vi "Test_Skew.vi"() -> ()   [LabVIEW 2020]
uses:
  <vilib>/vision/NI_Vision_Development_Module.lvlib
panel:
  in  "Sample":u16(ring) items=["Visualize", "Benchmark"]
  in  "Test Skewer":T1(ring)
  in  "Continious Skewing":bool
  in  "Calculation mode":enum16{"Single core", "2x cores", "4x cores"}(ring)
  out "Elapsed time [ms]":u32
  in  "Refresh Image":bool
  in  "Skew on X":bool
  in  "Share Angle":u16 max=89 step=1
  in  "stop":bool
  out "Image":T2(plugin-control)
  # "0, 1 ... 89"
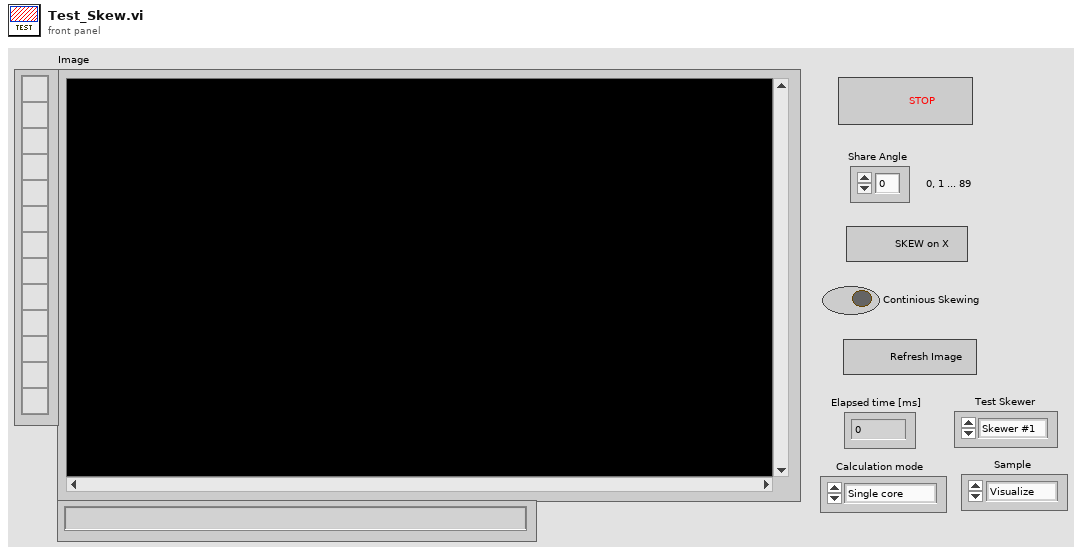
[diagram p1: front panel]
types:
  T1 = enum16{"Skewer #1", "Skewer #2", "Skewer #3", "Skewer #4", "Skewer #5"}
  T2 = typedef "IMAQ Image.ctl" = refnum<image>
  T3 = typedef "Image Type" = u32
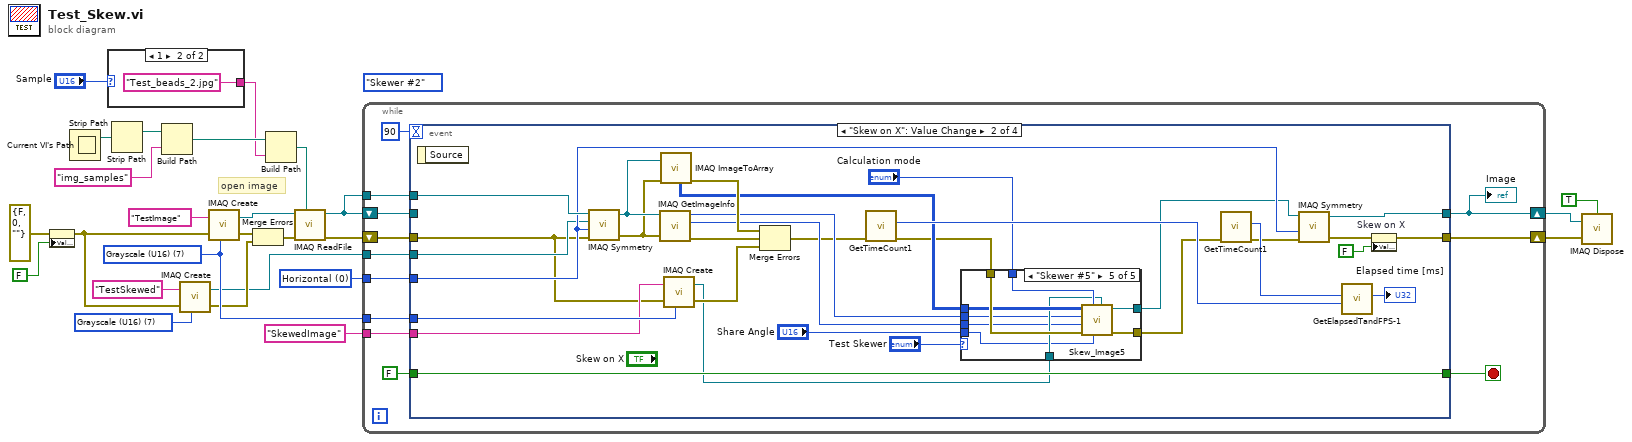
[diagram p0: block diagram]
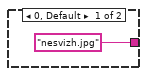
[diagram p2: hidden frame]
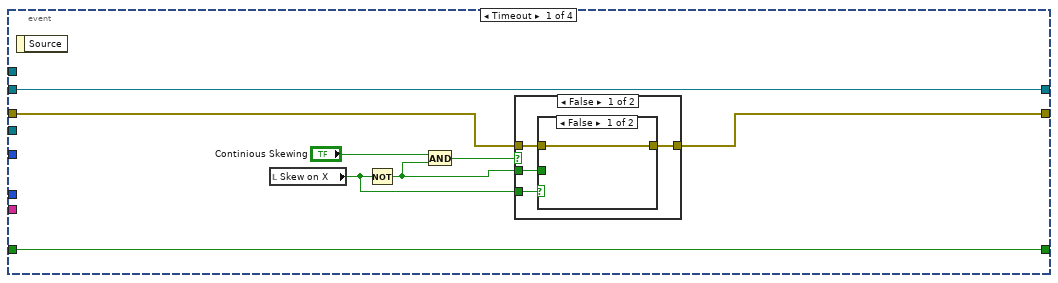
[diagram p3: hidden frame]
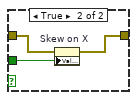
[diagram p4: hidden frame]
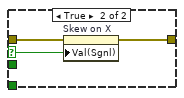
[diagram p5: hidden frame]
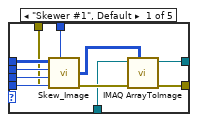
[diagram p6: hidden frame]
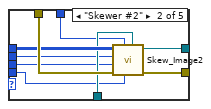
[diagram p7: hidden frame]
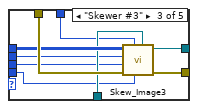
[diagram p8: hidden frame]
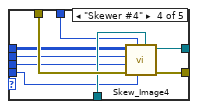
[diagram p9: hidden frame]
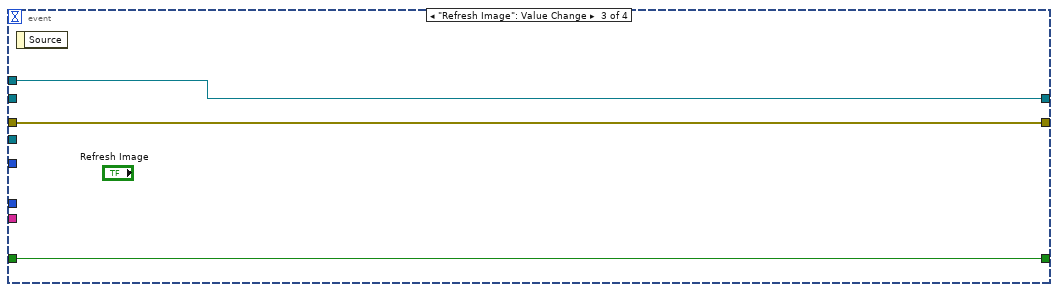
[diagram p10: hidden frame]
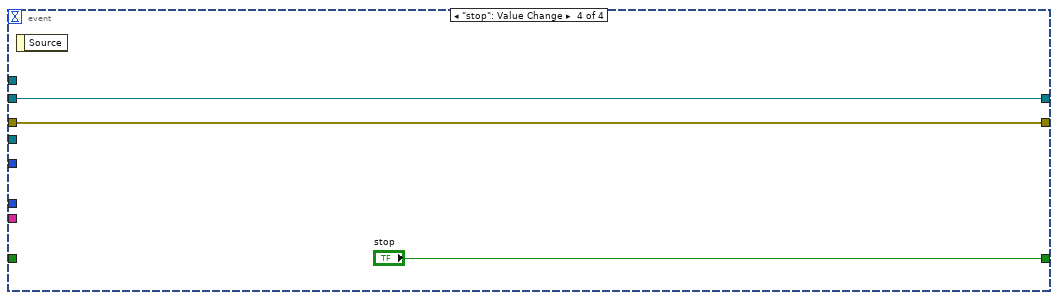
[diagram p11: hidden frame]
diagram:
  (unwired) enum16{"Skewer #1", "Skewer #2"}."Skewer #2"
  w11 = T3 7 items=["Grayscale (U8)", "Grayscale (I16)", "Grayscale (SGL)", "Complex (CSG)", "RGB (U32)", "HSL (U32)", "RGB (U64)", "Grayscale (U16)"] ("Image Type")
  w13 = u32 0 items=["Horizontal", "Vertical", "Central", "1st Diagonal", "2nd Diagonal"] ("Type of Symmetry")
  w17 = T3 7 items=["Grayscale (U8)", "Grayscale (I16)", "Grayscale (SGL)", "Complex (CSG)", "RGB (U32)", "HSL (U32)", "RGB (U64)", "Grayscale (U16)"] ("Image Type")
  # "open image"
  n1 = property on="Continious Skewing" class="Bool (strict)"(error in=errorcluster {"status"=FALSE, "code"=0, "source"=""} ("error in (no error)"), "Value"=FALSE ("Continious Skewing")) -> (error out=w4:errorcluster)  [unwired: 1 in, 1 out]
  n2 = Current VI's Path() -> (path=w27:path)
  n3 = Strip Path(path=w27) -> (stripped path=w23:path)  [unwired: 1 out]
  n4 = case shown="1" "Sample" {
    tunnel: ["nesvizh.jpg" ("name or relative path") "Test_beads_2.jpg" ("name or relative path")] -> w1
    frame 0, Default {
    }
    frame 1 {
    }
  }
  n5 = Strip Path(path=w23) -> (stripped path=w22:path)  [unwired: 1 out]
  n6 = Build Path(base path=w22, name or relative path="img_samples") -> (appended path=w20:path)
  n7 = call "IMAQ Create"("Image Name"="TestSkewed", "Image Type"=w11, "error in (no error)"=w4) -> ("New Image"=w7:T2, "error out"=w8:errorcluster)  [unwired: 2 in]
  n8 = call "IMAQ Create"("Image Name"="TestImage", "Image Type"=w17, "error in (no error)"=w4) -> ("New Image"=w24:T2, "error out"=w10:errorcluster)  [unwired: 2 in]
  n9 = Merge Errors(w10, w8) -> (w9:errorcluster)
  n10 = Build Path(base path=w20, name or relative path=w1) -> (appended path=w26:path)
  n11 = call "IMAQ ReadFile"("File Path"=w26, "error in (no error)"=w9, "Image"=w24) -> ("error out"=w19:errorcluster, "Image Out"=w15:T2)  [unwired: 4 in, 3 out]
  n12 = while {
    shift-right: [w39] -> w18
    shift-left: w19 -> [w40]
    tunnel: w17 -> [w35]
    shift-right: [w34] -> w14
    shift-left: w15 -> [w38]
    tunnel: w15 -> [w33]
    tunnel: w13 -> [w32]
    tunnel: w7 -> [w31]
    tunnel: "SkewedImage" ("Image Name") -> [w30]
    stop <- w36 stop-if-true
    n13 = event shown="[1] \"Skew on X\": Value Change" {
      selector: _ -> [_ _ _ _]
      dyn-events: _ -> [_ _ _ _]
      timeout: 90 -> [_ _ _ _]
      tunnel: w40 -> [w47 w67 w139 w143]
      tunnel: [w46 w72 w139 w143] -> w39
      tunnel: [w48 w91 w138 "stop"] -> w36
      tunnel: w38 -> [w49 _ _ w141]
      tunnel: [w49 w80 w140 w141] -> w34
      tunnel: FALSE ("stop") -> [w48 w91 w138 _]
      tunnel: w35 -> [_ w90 _ _]
      tunnel: w33 -> [_ w86 w140 _]
      tunnel: w32 -> [_ w83 _ _]
      tunnel: w31 -> [_ w82 _ _]
      tunnel: w30 -> [_ w81 _ _]
      event Timeout {
        n14 = event-data() -> ()  [unwired: 1 in, 1 out]
        n15 = local read "Skew on X"() -> (w43:bool)
        n16 = Not(x=w43) -> (.not. x?=w42:bool)
        n17 = And(x="Continious Skewing", y=w42) -> (x .and. y?=w44:bool)
        n18 = case shown="False" w44 {
          selector: w44 -> [_ w58]
          tunnel: w47 -> [w52 w60]
          tunnel: [w51 w59] -> w46
          tunnel: w43 -> [w53 _]
          tunnel: w42 -> [w50 _]
          frame False {
            n19 = case shown="False" w53 {
              tunnel: w52 -> [w54 w57]
              tunnel: [w54 w56] -> w51
              tunnel: w50 -> [_ w55]
              frame False {
              }
              frame True {
                n20 = property on="Skew on X" class="Bool (strict)"(error in=w57, "Value"=w55) -> (error out=w56:errorcluster)  [unwired: 1 in, 1 out]
              }
            }
          }
          frame True {
            n21 = property on="Skew on X" class="Bool (strict)"(error in=w60, "Val(Sgnl)"=w58) -> (error out=w59:errorcluster)  [unwired: 1 in, 1 out]
          }
        }
      }
      event "Skew on X": Value Change {
        n22 = event-data() -> ()  [unwired: 1 in, 1 out]
        n23 = call "IMAQ Symmetry"("error in (no error)"=w67, "Type of Symmetry"=w83, "Image Dst"=w82, "Image Src"=w86) -> ("error out"=w84:errorcluster, "Image Dst Out"=w85:T2)  [unwired: 1 in]
        n24 = call "IMAQ GetImageInfo"("error in (no error)"=w84, "Image"=w85) -> ("error out"=w89:errorcluster, "Y Resolution"=w73:i32, "X Resolution"=w74:i32)  [unwired: 2 in, 5 out]
        n25 = call "IMAQ ImageToArray"("error in (no error)"=w84, "Image"=w85) -> ("Image Pixels (U16)"=w75:u16[][], "error out"=w88:errorcluster)  [unwired: 2 in, 3 out]
        n26 = call "IMAQ Create"("Image Name"=w81, "Image Type"=w90, "error in (no error)"=w67) -> ("New Image"=w68:T2, "error out"=w87:errorcluster)  [unwired: 2 in]
        n27 = Merge Errors(w88, w89, w87) -> (w66:errorcluster)
        n28 = call "GetTimeCount1.vi"("error IN"=w66) -> ("error OUT"=w65:errorcluster, "[OUT] Timer Count"=w78:u32)  [unwired: 9 in]
        n29 = case shown="\"Skewer #5\"" "Test Skewer" {
          tunnel: "Share Angle" -> [w101 w104 w113 w120 w129]
          tunnel: w75 -> [w100 w109 w118 w126 w134]
          tunnel: w74 -> [w99 w106 w111 w122 w131]
          tunnel: w73 -> [w98 w105 w112 w121 w130]
          tunnel: "Calculation mode" -> [w97 w107 w116 w123 w133]
          tunnel: w65 -> [w96 w110 w119 w128 w137]
          tunnel: [w94 w102 w114 w124 w135] -> w64
          tunnel: [w93 w103 w115 w125 w136] -> w61
          tunnel: w68 -> [w92 w108 w117 w127 w132]
          frame "Skewer #1", Default {
            n30 = call "Skew_Image.vi"("[IN] Source Image U16"=w100, "[IN] X = Array cols"=w99, "[IN] Y = Array rows"=w98, "[IN] Share Angle"=w101, "[IN] Calculation mode"=w97) -> ("[OUT] Skewed Image"=w95:u16[][])  [unwired: 2 in]
            n31 = call "IMAQ ArrayToImage"("Image Pixels (U16)"=w95, "error in (no error)"=w96, "Image"=w92) -> ("error out"=w94:errorcluster, "Image Out"=w93:T2)  [unwired: 7 in]
          }
          frame "Skewer #2" {
            n32 = call "Skew_Image2.vi"("[IN] Skewed Image"=w108, "[IN] Share Angle"=w104, "[IN] Calculation mode"=w107, "error IN"=w110, "[IN] Y = Array rows"=w105, "[IN] X = Array cols"=w106, "[IN] Source Image U16"=w109) -> ("error OUT"=w102:errorcluster, "[OUT] Skewed Image"=w103:T2)  [unwired: 2 in]
          }
          frame "Skewer #3" {
            n33 = call "Skew_Image3.vi"("[IN] Skewed Image"=w117, "[IN] Share Angle"=w113, "[IN] Calculation mode"=w116, "error IN"=w119, "[IN] Y = Array rows"=w112, "[IN] X = Array cols"=w111, "[IN] Source Image U16"=w118) -> ("error OUT"=w114:errorcluster, "[OUT] Skewed Image"=w115:T2)  [unwired: 2 in]
          }
          frame "Skewer #4" {
            n34 = call "Skew_Image4.vi"("[IN] Skewed Image"=w127, "[IN] Share Angle"=w120, "[IN] Calculation mode"=w123, "error IN"=w128, "[IN] Y = Array rows"=w121, "[IN] X = Array cols"=w122, "[IN] Source Image U16"=w126) -> ("error OUT"=w124:errorcluster, "[OUT] Skewed Image"=w125:T2)  [unwired: 2 in]
          }
          frame "Skewer #5" {
            n35 = call "Skew_Image5.vi"("[IN] Skewed Image"=w132, "[IN] Share Angle"=w129, "[IN] Calculation mode"=w133, "error IN"=w137, "[IN] Y = Array rows"=w130, "[IN] X = Array cols"=w131, "[IN] Source Image U16"=w134) -> ("error OUT"=w135:errorcluster, "[OUT] Skewed Image"=w136:T2)  [unwired: 2 in]
          }
        }
        n36 = call "GetTimeCount1.vi"("error IN"=w64) -> ("error OUT"=w63:errorcluster, "[OUT] Timer Count"=w79:u32)  [unwired: 9 in]
        n37 = call "IMAQ Symmetry"("error in (no error)"=w63, "Type of Symmetry"=w83, "Image Src"=w61) -> ("error out"=w62:errorcluster, "Image Dst Out"=w80:T2)  [unwired: 2 in]
        n38 = call "GetElapsedTandFPS-1.vi"("[IN] Timer Count Before ALL [ms]"=w78, "[IN] Timer Count After ALL [ms]"=w79) -> ("[OUT] Elapsed time [ms]"=→"Elapsed time [ms]":u32)  [unwired: 3 in, 2 out]
        n39 = property on="Skew on X" class="Bool (strict)"(error in=w62, "Value"=FALSE ("Skew on X")) -> (error out=w72:errorcluster)  [unwired: 1 in, 1 out]
      }
      event "Refresh Image": Value Change {
        n40 = event-data() -> ()  [unwired: 1 in, 1 out]
      }
      event "stop": Value Change {
        n41 = event-data() -> ()  [unwired: 1 in, 1 out]
      }
    }
    "Image" <- w34
  }
  n42 = call "IMAQ Dispose"("All Images? (No)"=TRUE, "Image"=w14, "error in (no error)"=w18) -> ()  [unwired: 3 in, 1 out]
